vi "Get Colors.vi"(11 "Red Plugin in":refnum<class "Red Plugin.lvclass">) -> (3 "Color Box":u32(colorbox))   [LabVIEW 2020, in "Red Plugin.lvclass"]
uses:
  Red Plugin.lvclass
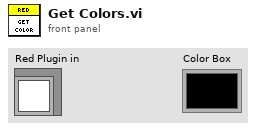
[diagram p1: front panel]
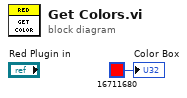
[diagram p0: block diagram]
diagram:
  "Color Box" <- u32 16711680 ("Color Box")
